vi "Test Caraya Init.vi"   [LabVIEW 2020]
uses:
  <vilib>/addons/_JKI Toolkits/Caraya/classes/Assert/Assert Equal Value_Variant.vi
  <vilib>/addons/_JKI Toolkits/Caraya/classes/Test/Test.lvclass
  <vilib>/addons/_JKI Toolkits/Caraya/classes/Assert/Assert.lvclass
  Libraries/Osciloscope/Osciloscope.lvlib
types:
  T1 = typedef "Osciloscope.lvlib/Broadcast Events--cluster.ctl" = cluster{"Module Did Init":refnum<user-event>, "Status Updated":refnum<user-event>, "Error Reported":refnum<user-event>, "Module Did Stop":refnum<user-event>, "Update Module Execution Status":refnum<user-event>, "OsciloscopesTypes":refnum<user-event>}
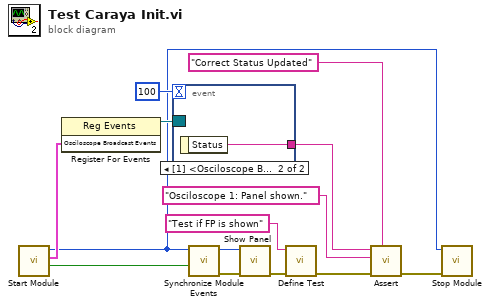
[diagram p0: block diagram]
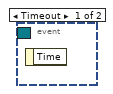
[diagram p2: hidden frame]
diagram:
  n1 = call "Start Module.vi"() -> ("Wait for Event Sync?"=w14:bool, "Osciloscope Broadcast Events"=w11:T1, "Module ID"=w1:i32)  [unwired: 8 in, 1 out]
  n2 = register-events(w11) -> (reference out=w10:refnum<event-registration>)  [unwired: 2 in, 1 out]
  n3 = event shown="[1] <Osciloscope Broadcast Events.Status Updated>: User Event" {
    selector: w10 -> [_ _]
    dyn-events: _ -> [_ _]
    timeout: 100 -> [_ _]
    tunnel: [_ w15] -> w6
    event Timeout {
      n4 = event-data() -> ()  [unwired: 1 in, 1 out]
    }
    event User Event {
      n5 = event-data() -> ("Status"=w15:string)  [unwired: 1 in]
    }
  }
  n6 = call "Synchronize Module Events.vi"("Wait for Event Sync?"=w14, "Module ID in"=w1) -> ("error out"=w12:errorcluster, "Module ID out"=w13:i32)  [unwired: 8 in]
  n7 = call "Show Panel.vi"("error in (no error)"=w12, "Module ID"=w13) -> ("error out"=w8:errorcluster)  [unwired: 9 in]
  n8 = call <vilib>:"Define Test.vi"("error in (no error)"=w8, "Label (VI Title)"="Test if FP is shown") -> ("error out"=w7:errorcluster)  [unwired: 9 in]
  n9 = call-poly <vilib>:"Assert.vi"("Label"="Correct Status Updated", "error in (no error)"=w7, "Y"="Osciloscope 1: Panel shown.", "X"=w6) -> ("error out"=w3:errorcluster)  [unwired: 7 in]
  n10 = call "Stop Module.vi"("error in (no error)"=w3, "Module ID"=w1) -> ()  [unwired: 9 in, 1 out]
